vi "Close Parent Window.vi"   [LabVIEW 2012]
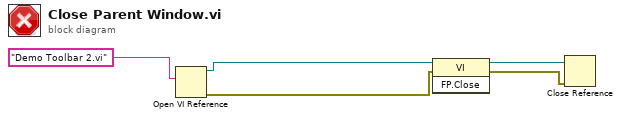
[diagram p0: block diagram]
diagram:
  n1 = Open VI Reference(vi path="Demo Toolbar 2.vi") -> (vi reference=w4:refnum<vi>, error out=w3:errorcluster)  [unwired: 1 in, 4 out]
  n2 = invoke class="VI" method="FP.Close"(reference=w4, error in=w3) -> (reference out=w5:refnum<vi>, error out=w2:errorcluster)  [unwired: 1 in, 1 out]
  n3 = Close Reference(reference=w5, error in (no error)=w2) -> ()  [unwired: 1 out]
